vi "TagBus_Read Table.vi"(10 "Index Array":i32[](array[numeric]), 11 "TagBus":refnum<class "TagBus.lvclass">) -> (2 "Value Array":dbl[](array[numeric]), 3 "TagBus out":refnum<class "TagBus.lvclass">)   [LabVIEW 2015, in "TagBus.lvclass"]
uses:
  TagBus.lvclass
  TagBus.lvclass/TagBus.ctl
  <vilib>/NI/Tag Bus/table/data polymorphs/read one/read Double.vi
  <vilib>/NI/Tag Bus/table/data table.lvlib
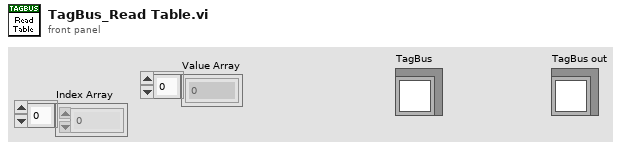
[diagram p1: front panel]
types:
  T1 = typedef "tag bus.lvlib/data table.lvlib/data table.ctl" = cluster{"Double":dbl[], "Single":sgl[], "I64":i64[], "I32":i32[], "I16":i16[], "I8":i8[], "U64":u64[], "U32":u32[], "U16":u16[], "U8":u8[], "Boolean":bool[], "String":string[], "Array of Double":cluster{"DBL Array":dbl[]}[], "Array of Single":cluster{"SGL Array":sgl[]}[], "Array of I64":cluster{"I64 Array":i64[]}[], "Array of I32":cluster{"I32 Array":i32[]}[], "Array of I16":cluster{"I16 Array":i16[]}[], "Array of I8":cluster{"I8 Array":i8[]}[], "Array of U64":cluster{"U64 Array":u64[]}[], "Array of U32":cluster{"U32 Array":u32[]}[], "Array of U16":cluster{"U16 Array":u16[]}[], "Array of U8":cluster{"U8 Array":u8[]}[], "Array of Boolean":cluster{"Boolean Array":bool[]}[], "Array of String":cluster{"String Array":string[]}[]}
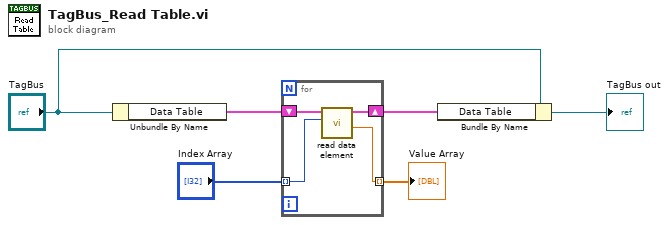
[diagram p0: block diagram]
diagram:
  n1 = Unbundle By Name("TagBus") -> ("Data Table"=w4:T1)
  n2 = for {
    tunnel: "Index Array" -> [w8] mode=indexing
    tunnel: [w7] -> w5 mode=indexing
    shift-right: [w9] -> w2
    shift-left: w4 -> [w10]
    n3 = call-poly <vilib>:"read data element.vi"("index"=w8, "data table in"=w10) -> ("value"=w7:dbl, "data table out"=w9:T1)  [unwired: 8 in]
  }
  "Value Array" <- w5
  n4 = Bundle By Name(cluster="TagBus", "Data Table"=w2) -> (→"TagBus out":refnum<class "TagBus.lvclass">)
